vi "scaninput.vi"(8 "error in (no error)":errorcluster, 11 "ZanCard in":refnum<class "ZanCard.lvclass">) -> (0 "error out":errorcluster, 3 "ZanCard out":refnum<class "ZanCard.lvclass">)   [LabVIEW 2019, in "ZanCard.lvclass"]
uses:
  ZanCard.lvclass
  ZanCard.lvclass/ZanCard.ctl
  LLB/zmotion/zaux/zauxdll.lvlib
panel:
  out "pistate out":u32
  in  "ionumfirst":i32
  in  "ionumend":i32=31
  out "function return":i32
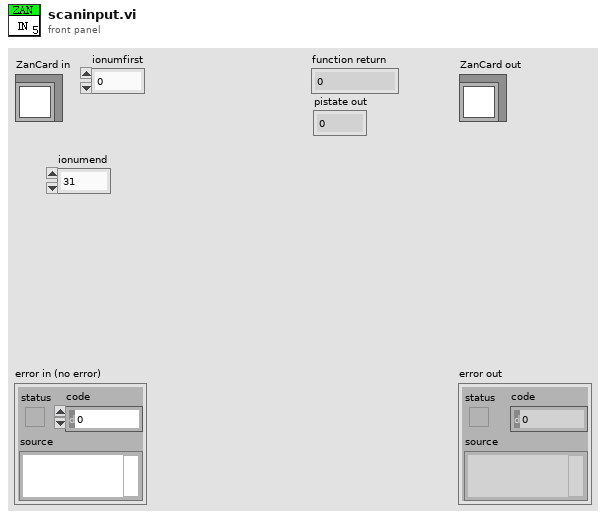
[diagram p1: front panel]
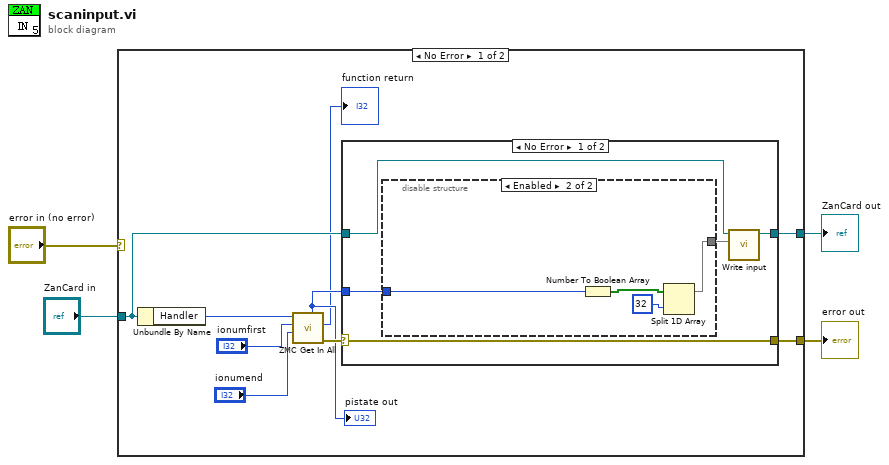
[diagram p0: block diagram]
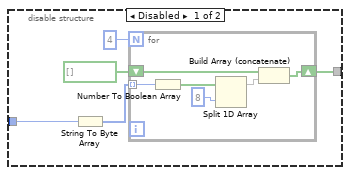
[diagram p2: hidden frame]
diagram:
  n1 = case shown="No Error" "error in (no error)" {
    selector: "error in (no error)" -> [_ w36]
    tunnel: "ZanCard in" -> [w12 w37]
    tunnel: [w11 w37] -> w2
    tunnel: [w9 w36] -> w1
    frame No Error {
      n2 = Unbundle By Name(w12) -> ("Handler"=w13:i32)
      n3 = call "ZMC Get In All.vi"("inumend"="ionumend", "inumfirst"="ionumfirst", "handle"=w13) -> ("error out"=w10:errorcluster, "function return"=→"function return":i32, "pistate out"=w6:u32)  [unwired: 5 in, 1 out]
      "pistate out" <- w6
      n4 = case shown="No Error" w10 {
        selector: w10 -> [w14 w34]
        tunnel: w6 -> [w18 _]
        tunnel: w12 -> [w17 w35]
        tunnel: [w15 w35] -> w11
        tunnel: [w14 w34] -> w9
        frame No Error {
          n5 = disable-structure shown="Enabled" {
            disable-tunnel: w18 -> [w23 w33]
            disable-tunnel: [w19 w30] -> w16
            frame Disabled {
              n6 = String To Byte Array(string=w23) -> (unsigned byte array=w22:u8[])
              n7 = for {
                N: 4 -> [_]
                tunnel: w22 -> [w29] mode=indexing
                shift-right: [w24] -> w19
                shift-left: bool[] [] -> [w25]
                n8 = Number To Boolean Array(number=w29) -> (Boolean array=w28:bool[])
                n9 = Split 1D Array(array=w28, index=8) -> (first subarray=w26:bool[])  [unwired: 1 out]
                n10 = Build Array (concatenate)(w25, w26) -> (w24:bool[])
              }
            }
            frame Enabled {
              n11 = Number To Boolean Array(number=w33) -> (Boolean array=w32:bool[])
              n12 = Split 1D Array(array=w32, index=32) -> (first subarray=w30:bool[])  [unwired: 1 out]
            }
          }
          n13 = call-dynamic "Write input.vi"("input"=w16, "IOCard in"=w17) -> ("IOCard out"=w15:refnum<class "ZanCard.lvclass">)  [unwired: 8 in, 1 out]
        }
        frame Error {
        }
      }
    }
    frame Error {
    }
  }
  "error out" <- w1
  "ZanCard out" <- w2
